vi "crio_RT_HX711_DMA.vi"() -> ()   [LabVIEW 2019]
uses:
  <vilib>/FPGAPlugInAG/cRIO-9074/niLvFpga_Open_cRIO-9074.vi
  <vilib>/rvi/interface/common/dynamic/niFpgaDynamicAddResources.vi
  <vilib>/Utility/error.llb/Error Cluster From Error Code.vi
  <vilib>/rvi/errors/niLvFpgaAdjustHostInterfaceError.vi
  <vilib>/FPGAPlugInAG/Dynamic/niLvFpga_Close_Dynamic.vi
  <vilib>/rvi/interface/nirviOpenFPGA/nirviOpenFPGA.xnode
  FPGA Bitfiles/gpass2_FPGATarget2_crioFPGALAC_7QpNv7lccB4.lvbitx
  crio_FPGA_LAC_HX711.vi
  <vilib>/rvi/interface/nirviReadWriteControl/nirviReadWriteControl.xnode
  <vilib>/rvi/interface/nirviMethod/nirviMethod.xnode
  <vilib>/rvi/interface/nirviCloseFPGA/nirviCloseFPGA.xnode
  NiFpgaLv.dll
  <vilib>/rvi/interface/Simulation/niFpgaSimulationCallBeginRW.vi
  <vilib>/ptbypt/NI_PtbyPt.lvlib
  <vilib>/FPGAPlugInAG/Dynamic/niLvFpga_ReadFifo_Dynamic.vi
  <vilib>/rvi/errors/niLvFpgaMergeErrorWithErrorCode.vi
panel:
  out "Raw Data":i32(graph)
  in  "stop":bool
  out "HX711 Raw Data":i32
  in  "Gain/ChannelSelect":T1(ring)=enum."Channel A/Gain 64"
  out "FIFO Data":i32(graph)
  out "Computed Bias":dbl(graph)
  out "Offsetted Data":dbl(graph)
  out "Computed Bias":dbl format="%0.2f"
  in  "Number of Samples for Offset Computation":i32=100
  in  "Offset Bias":bool
  out "Offsetted Data":dbl
  in  "FIFO Element Threshold":u32
  out "HX711 FIFO Data":i32[](array[numeric])
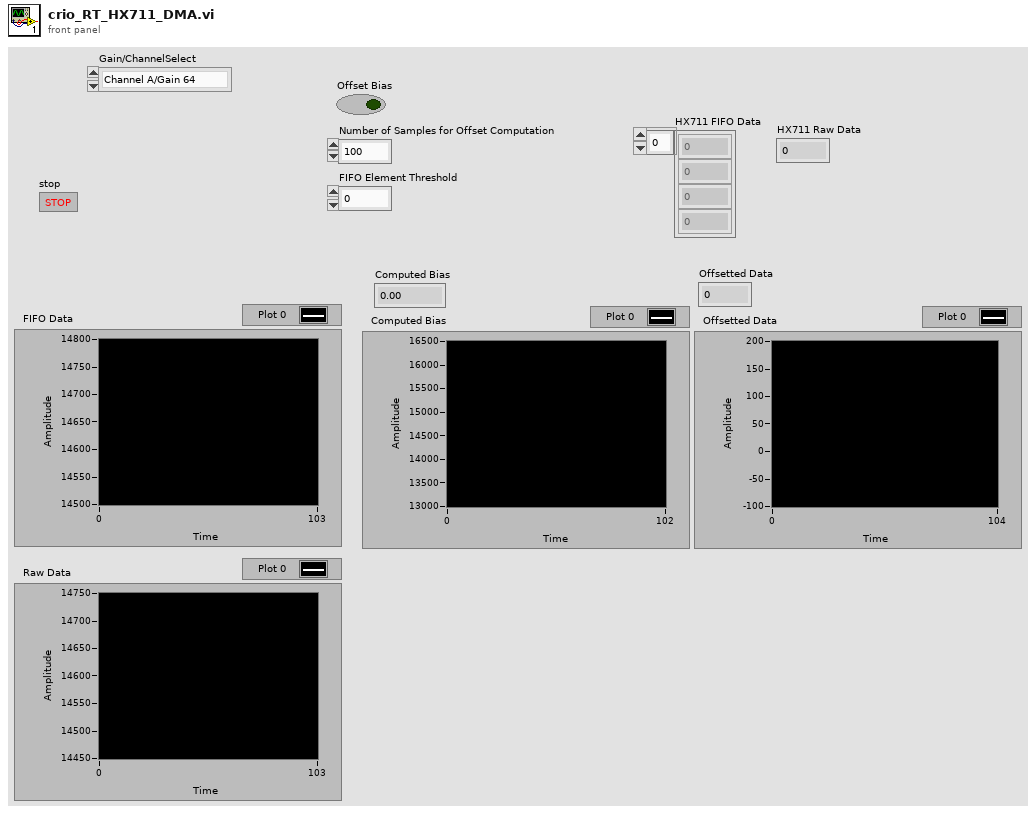
[diagram p1: front panel]
types:
  T1 = enum16{"Channel A/Gain 128", "Channel A/Gain 64", "Channel B/Gain 32"}
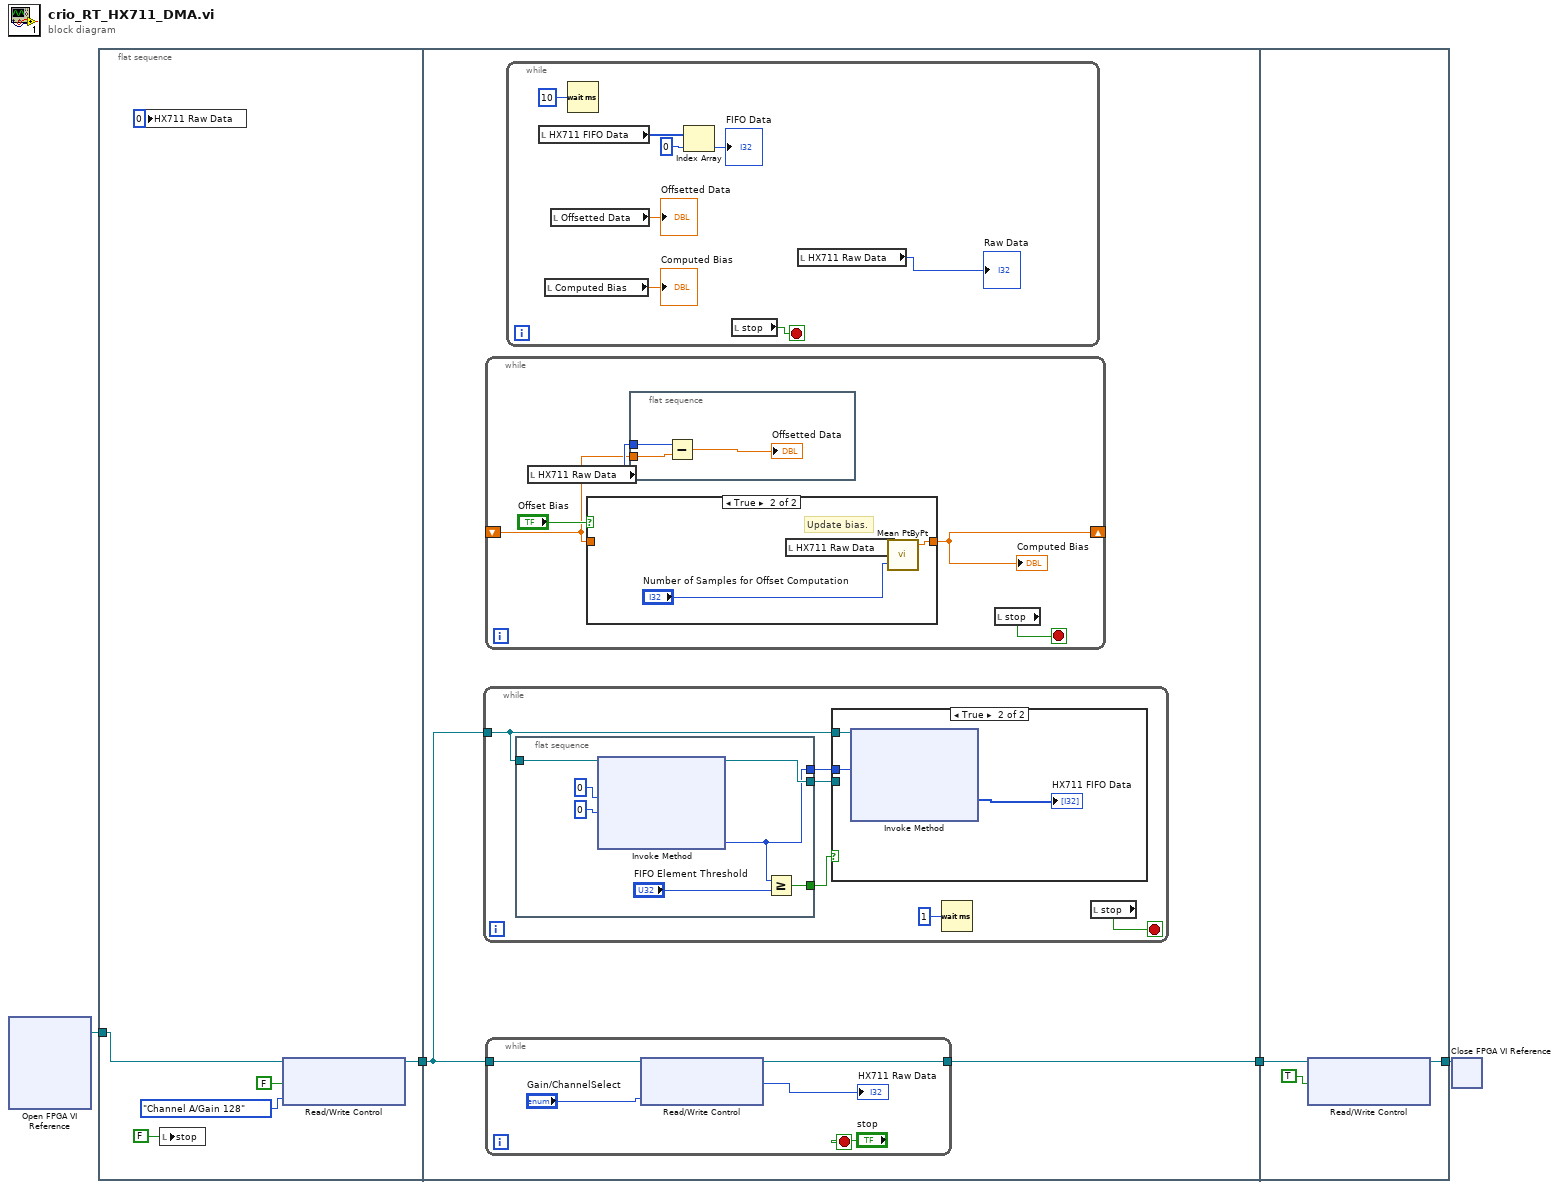
[diagram p0: block diagram]
diagram:
  n1 = xnode "Open FPGA VI Reference"() -> ("FPGA VI Reference Out"=w1:refnum<k20>)  [unwired: 2 in, 1 out]
  n2 = flat-sequence {
    tunnel: [w9] -> w4
    tunnel: w1 -> [w5]
    tunnel: w4 -> [w11]
    tunnel: [w12] -> w3
    tunnel: w3 -> [w55]
    tunnel: [w54] -> w2
    frame #0 {
      n3 = local write "HX711 Raw Data"(0 ("Data")) -> ()
      n4 = local write "stop"(FALSE ("stop")) -> ()
      n5 = xnode "Read/Write Control"("FPGA VI Reference In"=w5, "stop"=FALSE, "Gain/ChannelSelect"=T1."Channel A/Gain 128") -> ("FPGA VI Reference Out"=w9:refnum<k20>)  [unwired: 1 in, 1 out]
    }
    frame #1 {
      n6 = while {
        tunnel: w11 -> [w18]
        stop <- w16 stop-if-true
        n7 = flat-sequence {
          tunnel: w18 -> [w28]
          tunnel: [w26] -> w17
          tunnel: [w25] -> w15
          tunnel: [w24] -> w14
          frame #0 {
            n8 = xnode "Invoke Method"("FPGA VI Reference In"=w28, "Number of Elements"=0 ("Timeout (ms)"), "Timeout (ms)"=u32 0 ("Number of Elements")) -> ("FPGA VI Reference Out"=w26:refnum<k20>, "Elements Remaining"=w24:u32)  [unwired: 1 in, 2 out]
            n9 = Greater Or Equal?(x=w24, y="FIFO Element Threshold") -> (x >= y?=w25:bool)
          }
        }
        n10 = case shown="True" w15 {
          tunnel: w18 -> [_ w21]
          tunnel: w17 -> [_ _]
          tunnel: w14 -> [_ w20]
          frame False {
          }
          frame True {
            n11 = xnode "Invoke Method"("FPGA VI Reference In"=w21, "Number of Elements"=w20) -> ("Data"=→"HX711 FIFO Data":i32[])  [unwired: 2 in, 3 out]
          }
        }
        n12 = Wait (ms)(milliseconds to wait=u32 1) -> ()  [unwired: 1 out]
        n13 = local read "stop"() -> (w16:bool)
      }
      n14 = while {
        shift-right: [w31] -> _
        shift-left: _ -> [w29]
        stop <- w33 stop-if-true
        n15 = local read "HX711 Raw Data"() -> (w30:i32)
        n16 = case shown="True" "Offset Bias" {
          tunnel: [w37 w39] -> w31
          tunnel: w29 -> [w37 _]
          frame False {
            # "Stick with latest bias."
          }
          frame True {
            # "Update bias."
            n17 = local read "HX711 Raw Data"() -> (w40:i32)
            n18 = call <vilib>:"Mean PtByPt.vi"("x"=w40, "sample length"="Number of Samples for Offset Computation") -> ("mean"=w39:dbl)  [unwired: 2 in, 1 out]
          }
        }
        "Computed Bias" <- w31
        n19 = flat-sequence {
          tunnel: w30 -> [w36]
          tunnel: w29 -> [w35]
          frame #0 {
            n20 = Subtract(x=w36, y=w35) -> (x-y=→"Offsetted Data":dbl)
          }
        }
        n21 = local read "stop"() -> (w33:bool)
      }
      n22 = while {
        tunnel: w11 -> [w53]
        tunnel: [w50] -> w12
        stop <- "stop" stop-if-true
        n23 = xnode "Read/Write Control"("FPGA VI Reference In"=w53, "Gain/ChannelSelect"="Gain/ChannelSelect") -> ("FPGA VI Reference Out"=w50:refnum<k20>, "Data"=→"HX711 Raw Data":i32)  [unwired: 1 in, 1 out]
      }
      n24 = while {
        stop <- w48 stop-if-true
        n25 = local read "HX711 FIFO Data"() -> (w44:i32[])
        n26 = local read "Computed Bias"() -> (→"Computed Bias":dbl)
        n27 = local read "Offsetted Data"() -> (→"Offsetted Data":dbl)
        n28 = Wait (ms)(milliseconds to wait=u32 10) -> ()  [unwired: 1 out]
        n29 = Index Array(array=w44, index=0) -> (element=→"FIFO Data":i32)
        n30 = local read "stop"() -> (w48:bool)
        n31 = local read "HX711 Raw Data"() -> (→"Raw Data":i32)
      }
    }
    frame #2 {
      n32 = xnode "Read/Write Control"("FPGA VI Reference In"=w55, "stop"=TRUE) -> ("FPGA VI Reference Out"=w54:refnum<k20>)  [unwired: 2 in, 1 out]
    }
  }
  n33 = xnode "Close FPGA VI Reference"("FPGA VI Reference In"=w2) -> ()  [unwired: 1 in, 1 out]
